vi "Daemon Async.vi"(10 "Close Notifier":refnum<notifier>, 11 "Session Notifier":refnum<notifier>) -> ()   [LabVIEW 2020, in "Conditu2.lvlib" / "Unit Of Work Session.lvclass"]
uses:
  Unit Of Work Session.lvclass
  Unit Of Work Session.lvclass/Unit Of Work Session.ctl
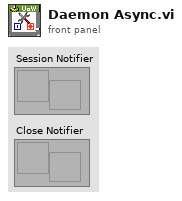
[diagram p1: front panel]
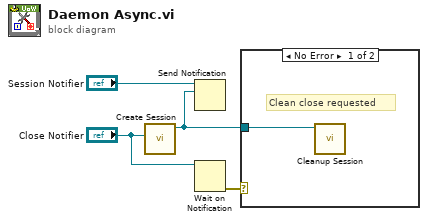
[diagram p0: block diagram]
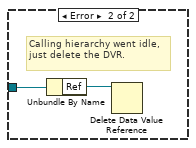
[diagram p2: hidden frame]
diagram:
  n1 = call "Create Session.vi"("Close Notifier"="Close Notifier") -> ("Unit Of Work out"=w1:refnum<class "Unit Of Work Session.lvclass">)  [unwired: 9 in, 1 out]
  n2 = Send Notification(notification=w1, notifier="Session Notifier") -> ()  [unwired: 1 in, 2 out]
  n3 = Wait on Notification(notifier="Close Notifier") -> (error out=w2:errorcluster)  [unwired: 3 in, 3 out]
  n4 = case shown="No Error" w2 {
    tunnel: w1 -> [w5 w7]
    frame No Error {
      # "Clean close requested"
      n5 = call "Cleanup Session.vi"("Unit Of Work in"=w5) -> ()  [unwired: 10 in, 1 out]
    }
    frame Error {
      # "Calling hierarchy went idle, just delete the DVR."
      n6 = Unbundle By Name(w7) -> ("Ref"=w6:refnum<data-value>)
      n7 = Delete Data Value Reference(data value reference=w6) -> ()  [unwired: 1 in, 2 out]
    }
  }
